vi "Set Needle Configuration.vi"(8 "error in (no error)":errorcluster, 10 "Needle Configuration in":bool, 11 "Item Ref in":T1 format="%.0x") -> (0 "error out":errorcluster, 2 "Needle Configuration out":bool, 3 "Item Ref out":T1 format="%.0x")   [LabVIEW 2011, in "Meter Detection Custom Device.lvlib"]
uses:
  Meter Detection Custom Device.lvlib
  <vilib>/NI Veristand/Custom Device API/Custom Device Item Ref.ctl
  Meter Detection Global Variable.vi
  <vilib>/NI Veristand/Custom Device API/Set Item Property (Boolean).vi
  <vilib>/NI Veristand/Custom Device API/Custom Device API.lvlib
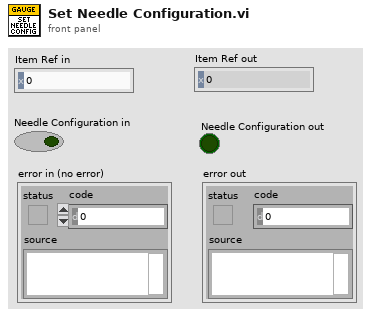
[diagram p1: front panel]
types:
  T1 = typedef "Custom Device API.lvlib/Custom Device Item Ref.ctl" = u64
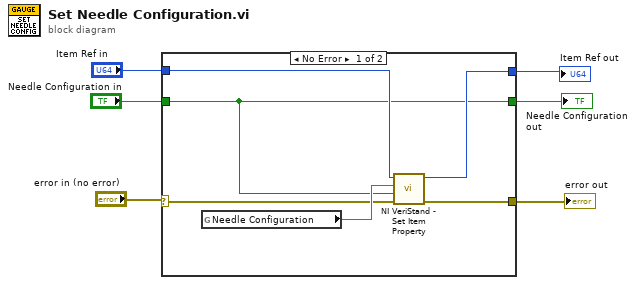
[diagram p0: block diagram]
diagram:
  n1 = case shown="No Error" "error in (no error)" {
    selector: "error in (no error)" -> [w8 w13]
    tunnel: [w7 w14] -> w6
    tunnel: "Needle Configuration in" -> [w7 w14]
    tunnel: [w11 w13] -> w4
    tunnel: "Item Ref in" -> [w10 w15]
    tunnel: [w9 w15] -> w2
    frame No Error {
      n2 = global read "Meter Detection Global Variable.vi" "Needle Configuration"() -> (w12:string)
      n3 = call-poly <vilib>:"NI VeriStand - Set Item Property.vi"("error in (no error)"=w8, "Value"=w7, "Property Name"=w12, "Item Ref in"=w10) -> ("error out"=w11:errorcluster, "Item Ref out"=w9:T1)  [unwired: 5 in, 1 out]
    }
    frame Error {
    }
  }
  "Needle Configuration out" <- w6
  "error out" <- w4
  "Item Ref out" <- w2
